vi "OpenNetworkStreamReader.vi"(7 "reader buffer size":i32, 8 "error in (no error)":errorcluster, 9 "writer url":string, 10 "reader name":string, 11 "NetworkStreamReader in":refnum<class "NetworkStreamReader.lvclass">) -> (0 "error out":errorcluster, 2 "Reader Endpoint":refnum<k21>, 3 "NetworkStreamReader out":refnum<class "NetworkStreamReader.lvclass">)   [LabVIEW 2011, in "NetworkStreamReader.lvclass"]
doc: "Opens a network stream reader endpoint. This VI persistently tries to open the connection until it is successful or the e-stop is triggered."
uses:
  NetworkStreamReader.lvclass
  Shared/message.ctl
  NetworkStreamReader.lvclass/NetworkStreamReader.ctl
  2-Think/2 Globals/2 Global.vi
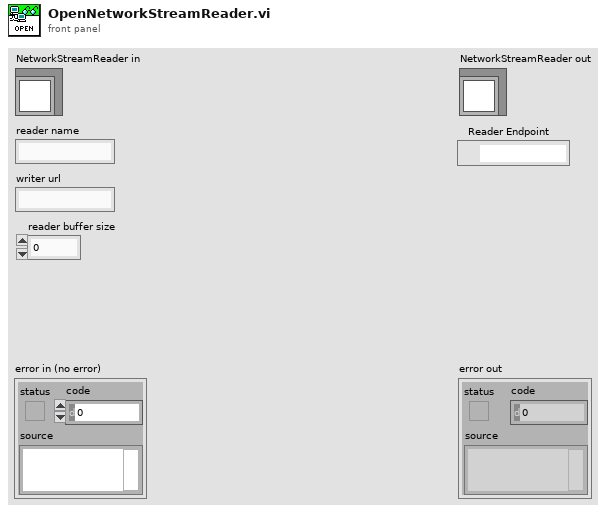
[diagram p1: front panel]
types:
  T1 = typedef "message.ctl" = cluster{"Data":variant, "Time since start (s)":dbl}
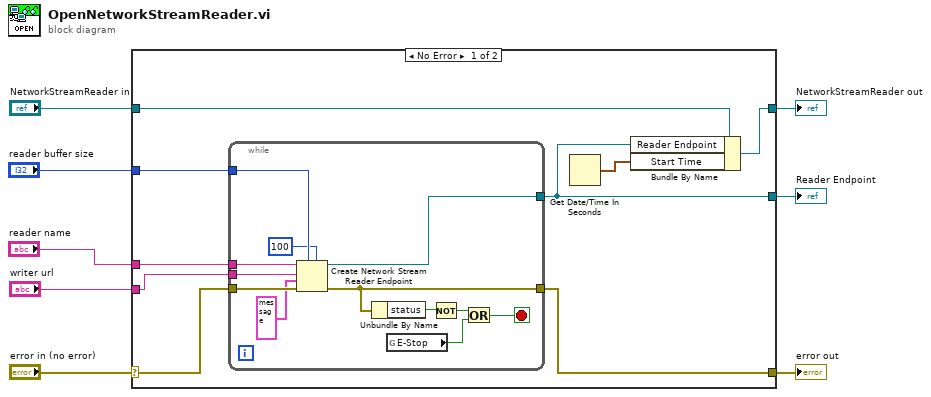
[diagram p0: block diagram]
diagram:
  n1 = case shown="No Error" "error in (no error)" {
    selector: "error in (no error)" -> [w17 w31]
    tunnel: [w15 w31] -> w7
    tunnel: [w13 w30] -> w5
    tunnel: "NetworkStreamReader in" -> [w14 w30]
    tunnel: "reader buffer size" -> [w16 _]
    tunnel: "reader name" -> [w12 _]
    tunnel: "writer url" -> [w11 _]
    tunnel: [w10 _] -> w1
    frame No Error {
      n2 = while {
        tunnel: w17 -> [w29]
        tunnel: w16 -> [w28]
        tunnel: [w23] -> w15
        tunnel: w12 -> [w27]
        tunnel: w11 -> [w26]
        tunnel: [w19] -> w10
        stop <- w20 stop-if-true
        n3 = Create Network Stream Reader Endpoint(5:100 ("timeout in ms (-1)"), 7:w28, 8:w29, 9:T1 {"Data"=variant, "Time since start (s)"=0.0} ("variant"), 10:w26, 11:w27) -> (0:w23:errorcluster, 3:w19:refnum<k21>)
        n4 = Unbundle By Name(w23) -> ("status"=w22:bool)
        n5 = global read "2 Global.vi" "E-Stop"() -> (w18:bool)
        n6 = Not(x=w22) -> (.not. x?=w21:bool)
        n7 = Or(x=w21, y=w18) -> (x .or. y?=w20:bool)
      }
      n8 = Get Date/Time In Seconds() -> (seconds since 1Jan1904=w9:timestamp)
      n9 = Bundle By Name(cluster=w14, "Reader Endpoint"=w10, "Start Time"=w9) -> (w13:refnum<class "NetworkStreamReader.lvclass">)
    }
    frame Error {
    }
  }
  "error out" <- w7
  "NetworkStreamReader out" <- w5
  "Reader Endpoint" <- w1
